vi "GDS_MO_GetEnergy_TEST.vi"() -> ()   [LabVIEW 2015]
uses:
  SES_1.3.1-r26_SES100/dll/MonoHW_Dummy.dll
panel:
  out "error out":errorcluster
  out "return type":i8
  out "AEnergy_Dummy":dbl=750.0
  # "GetEnergy"
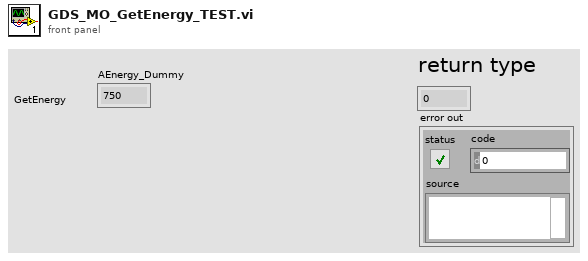
[diagram p1: front panel]
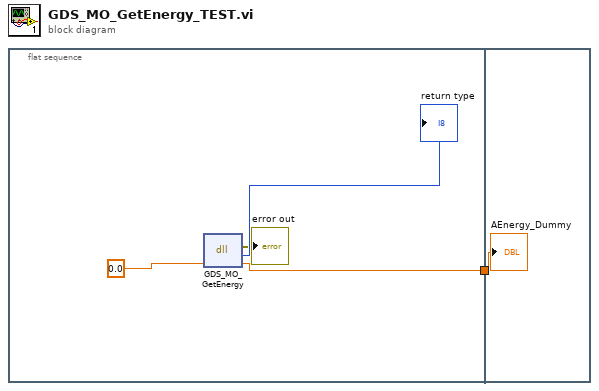
[diagram p0: block diagram]
diagram:
  n1 = flat-sequence {
    tunnel: [w3] -> w1
    tunnel: w1 -> [w6]
    frame #0 {
      n2 = dll-call lib="S:/SES_1.3.1-r26_SES100/dll/MonoHW_Dummy.dll" fn="GDS_MO_GetEnergy"("arg1"=0.0) -> (error out=→"error out":errorcluster, "return type"=→"return type":i16, "arg1"=w3:dbl)  [unwired: 3 in, 1 out]
    }
    frame #1 {
      "AEnergy_Dummy" <- w6
    }
  }
